vi "Assert Test In Library.vi"(8 "error in (no error)":errorcluster) -> (0 "error out":errorcluster)   [LabVIEW 2013, in "test-lvlib.lvlib" / "test-nested-lvlib.lvlib"]
uses:
  test-nested-lvlib.lvlib
  classes/Assert/Assert.lvclass
  classes/Test/Test.lvclass
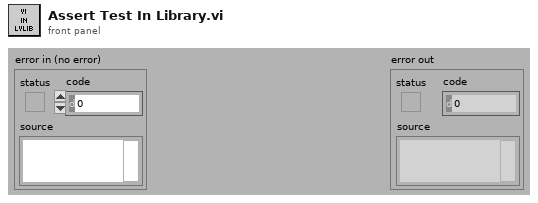
[diagram p1: front panel]
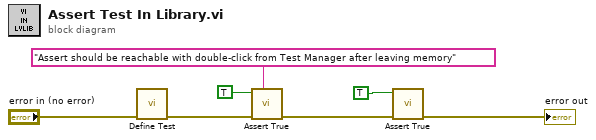
[diagram p0: block diagram]
diagram:
  n1 = call "Define Test.vi"("error in (no error)"="error in (no error)") -> ("error out"=w4:errorcluster)  [unwired: 10 in]
  n2 = call "Assert True.vi"("Label"="Assert should be reachable with double-click from Test Manager after leaving memory", "error in (no error)"=w4, "True?"=TRUE) -> ("error out"=w3:errorcluster)  [unwired: 8 in]
  n3 = call "Assert True.vi"("error in (no error)"=w3, "True?"=TRUE) -> ("error out"=→"error out":errorcluster)  [unwired: 9 in]
